vi "Fotemp.vi"() -> ()   [LabVIEW 2020]
uses:
  <vilib>/Instr/_visa.llb/VISA Configure Serial Port (Instr).vi
panel:
  in  "Periodo de muestreo (ms)":u32
  out "Temperatura / t":cluster{dbl[], dbl[]}(graph)
  out "Marca de tiempo":dbl
  out "Temperatura":dbl
  in  "Canal (1 - 4)":i32
  in  "?":bool
  in  "Puerto FOTEMP":refnum<visa-resource-name>
  out "Error":errorcluster
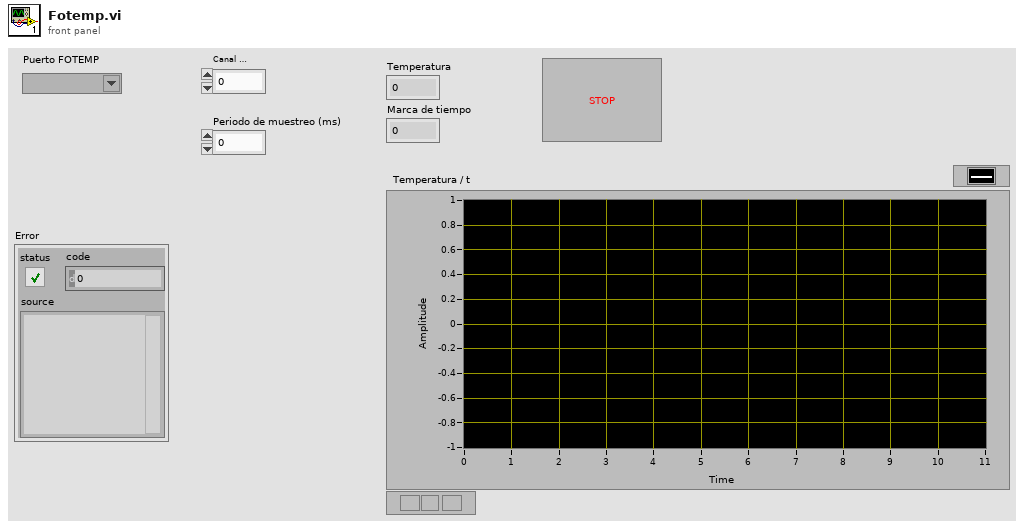
[diagram p1: front panel]
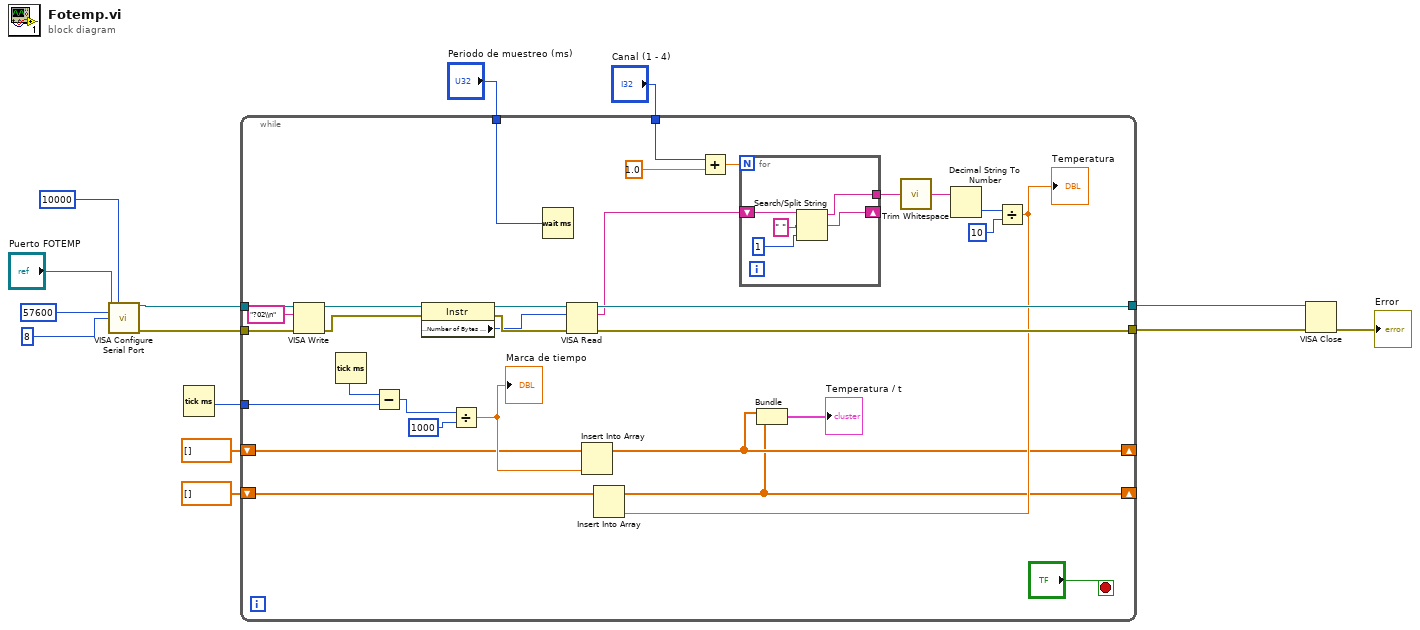
[diagram p0: block diagram]
diagram:
  n1 = call-poly "VISA Configure Serial Port"("VISA resource name"="Puerto FOTEMP", "timeout (10sec)"=u32 10000, "baud rate (57600)"=u32 57600 ("baud rate (9600)"), "data bits (8)"=u16 8) -> ("VISA resource name out"=w10:refnum<visa-resource-name>, "error out"=w9:errorcluster)  [unwired: 10 in]
  n2 = Tick Count (ms)() -> (millisecond timer value=w5:u32)
  n3 = while {
    tunnel: w10 -> [w45]
    tunnel: w9 -> [w44]
    tunnel: [w39] -> w8
    tunnel: [w37] -> w7
    tunnel: "Canal (1 - 4)" -> [w31]
    tunnel: w5 -> [w27]
    shift-right: [w17] -> _
    shift-left: dbl[] [] -> [w20]
    shift-right: [w18] -> _
    shift-left: dbl[] [] -> [w21]
    tunnel: "Periodo de muestreo (ms)" -> [w15]
    stop <- "?" stop-if-true
    n4 = VISA Write(VISA resource name=w45, write buffer="?02\\n", error in (no error)=w44) -> (VISA resource name out=w43:refnum<visa-resource-name>, error out=w41:errorcluster)  [unwired: 1 out]
    n5 = Tick Count (ms)() -> (millisecond timer value=w28:u32)
    n6 = Subtract(x=w28, y=w27) -> (x-y=w25:u32)
    n7 = property class="Instr"(reference=w43, error in=w41) -> (reference out=w42:refnum<visa-resource-name>, error out=w40:errorcluster, "Serial Settings:Number of Bytes at Serial Port"=w38:u32)
    n8 = Divide(x=w25, y=u32 1000) -> (x/y=w22:dbl)
    "Marca de tiempo" <- w22
    n9 = Wait (ms)(milliseconds to wait=w15) -> ()  [unwired: 1 out]
    n10 = VISA Read(VISA resource name=w42, byte count=w38, error in (no error)=w40) -> (VISA resource name out=w39:refnum<visa-resource-name>, read buffer=w34:string, error out=w37:errorcluster)  [unwired: 1 out]
    n11 = Insert Into Array(array=w21, new element=w22) -> (w18:dbl[])  [unwired: 1 in]
    n12 = Add(x=w31, y=1.0) -> (x+y=w32:dbl)
    n13 = for {
      N: w32 -> [_]
      shift-right: [w48] -> _
      shift-left: w34 -> [w49]
      tunnel: [w47] -> w30
      n14 = Search/Split String(string=w49, search string/char (-)=" ", offset (0)=1) -> (substring before match=w47:string, match + rest of string=w48:string)  [unwired: 1 out]
    }
    n15 = call <vilib>:"Trim Whitespace.vi"("string"=w30) -> ("trimmed string"=w29:string)  [unwired: 1 in]
    n16 = Decimal String To Number(string=w29) -> (number=w26:i32)  [unwired: 2 in, 1 out]
    n17 = Divide(x=w26, y=10 ("x")) -> (x/y=w19:dbl)
    "Temperatura" <- w19
    n18 = Insert Into Array(array=w20, new element=w19) -> (w17:dbl[])  [unwired: 1 in]
    n19 = Bundle(w18, w17) -> (→"Temperatura / t":cluster{dbl[], dbl[]})  [unwired: 1 in]
  }
  n20 = VISA Close(VISA resource name=w8, error in (no error)=w7) -> (error out=→"Error":errorcluster)
